vi "Print XML Recursive Priv.vi"(0 "Tree Dictionary In":variant, 1 "Recursion Level":i32, 2 "Data Types Dict":variant, 7 "Child IDs":string[](array[string]), 11 "error in":errorcluster, 12 "Include Type Attribute":bool=TRUE) -> (4 "Tree Dictionary Out":variant, 8 "XML String":string, 15 "error out":errorcluster)   [LabVIEW 2020, in "NI_VIAnCFGDataStructure.lvlib" / "Tree.lvclass"]
uses:
  <vilib>/addons/analyzer/VIAnCFGDataStructure/Tree Manager/Tree.lvclass
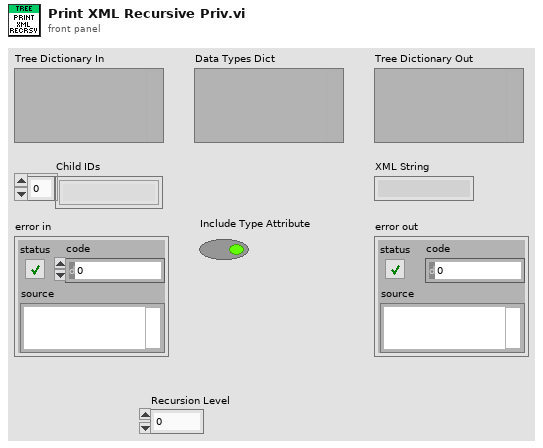
[diagram p1: front panel]
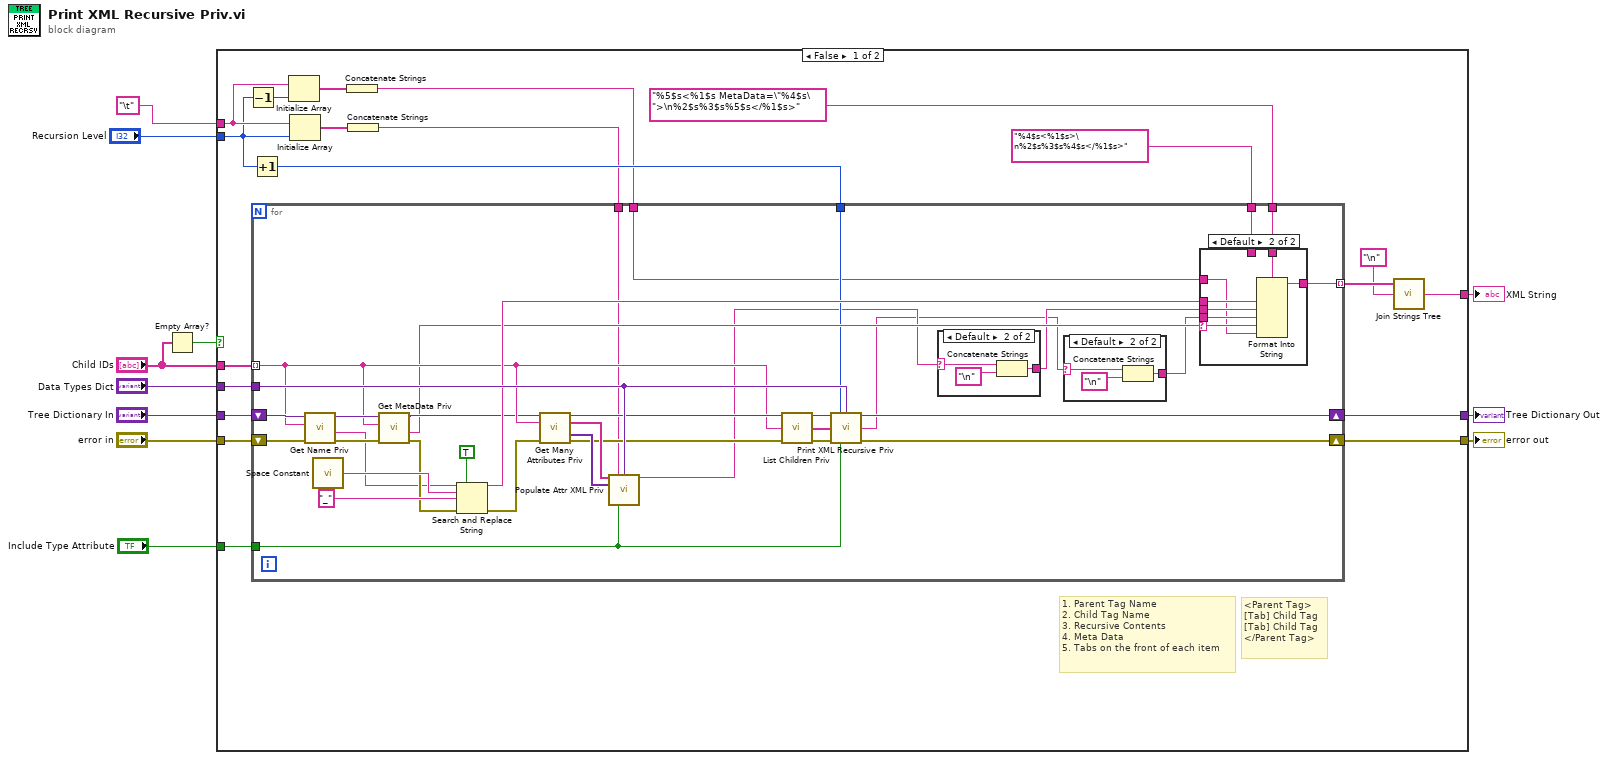
[diagram p0: block diagram]
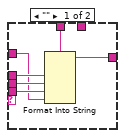
[diagram p4: hidden frame]
diagram:
  n1 = Empty Array?(array="Child IDs") -> (empty?=w1:bool)
  n2 = case shown="False" w1 {
    tunnel: [w31 w88] -> w11
    tunnel: "error in" -> [w30 w88]
    tunnel: "Tree Dictionary In" -> [w29 w89]
    tunnel: [w28 w89] -> w8
    tunnel: "Data Types Dict" -> [w27 _]
    tunnel: "Include Type Attribute" -> [w23 _]
    tunnel: "\t" -> [w15 _]
    tunnel: "Recursion Level" -> [w13 _]
    tunnel: [w19 _] -> w3
    tunnel: "Child IDs" -> [w17 _]
    frame False {
      # "<Parent Tag>\n[Tab] Child Tag\n[Tab] Child Tag\n</Parent Tag>"
      # "1. Parent Tag Name\n2. Child Tag Name\n3. Recursive Contents\n4. Meta Data\n5. Tabs on the front of each item"
      n3 = Decrement(x=w13) -> (x-1=w14:i32)
      n4 = Increment(x=w13) -> (x+1=w21:i32)
      n5 = Initialize Array(w15, w14) -> (w16:string[])
      n6 = Initialize Array(w15, w13) -> (w22:string[])
      n7 = Concatenate Strings(w16) -> (w12:string)
      n8 = Concatenate Strings(w22) -> (w20:string)
      n9 = for {
        tunnel: w17 -> [w47] mode=indexing
        shift-right: [w63] -> w28
        shift-left: w29 -> [w66]
        shift-right: [w53] -> w31
        shift-left: w30 -> [w65]
        tunnel: w27 -> [w61]
        tunnel: [w40] -> w26 mode=indexing
        tunnel: "%5$s<%1$s MetaData=\"%4$s\">\n%2$s%3$s%5$s</%1$s>" ("format string") -> [w43]
        tunnel: "%4$s<%1$s>\n%2$s%3$s%4$s</%1$s>" ("format string") -> [w42]
        tunnel: w23 -> [w41]
        tunnel: w21 -> [w39]
        tunnel: w20 -> [w32]
        tunnel: w12 -> [w33]
        n10 = call <vilib>:"Get Name Priv.vi"("error in"=w65, "Unique ID"=w47, "Tree Dictionary"=w66) -> ("error out"=w48:errorcluster, "Name"=w37:string, "Tree Dictionary Out"=w49:variant)  [unwired: 6 in]
        n11 = call <vilib>:"Space Constant.vi"() -> ("String"=w58:string)
        n12 = call <vilib>:"Get MetaData Priv.vi"("error in"=w48, "Unique ID"=w47, "Tree Dictionary"=w49) -> ("error out"=w45:errorcluster, "MetaData"=w44:string, "Tree Dictionary Out"=w46:variant)  [unwired: 6 in]
        n13 = Search and Replace String(replace all?=TRUE ("replace all? (F)"), input string=w37, search string=w58, replace string="_", error in=w45) -> (result string=w55:string, error out=w54:errorcluster)  [unwired: 3 in, 2 out]
        n14 = call <vilib>:"Get Many Attributes Priv.vi"("Tree Dictionary In"=w46, "Unique ID"=w47, "error in"=w54) -> ("Tree Dictionary Out"=w59:variant, "Attribute Names"=w52:string[], "Attribute Values"=w51:variant[], "error out"=w50:errorcluster)  [unwired: 8 in, 1 out]
        n15 = call <vilib>:"Populate Attr XML Priv.vi"("Attribute Names"=w52, "Tab String"=w32, "Data Types Dict"=w61, "Attribute Values"=w51, "Include Type Attribute"=w41) -> ("Attr XML String"=w38:string)  [unwired: 10 in]
        n16 = call <vilib>:"List Children Priv.vi"("Tree Dictionary"=w59, "Parent ID"=w47, "Error In"=w50) -> ("Tree Dictionary Out"=w64:variant, "Child IDs"=w62:string[], "Error Out"=w60:errorcluster)  [unwired: 10 in]
        n17 = call <vilib>:"Print XML Recursive Priv.vi"("Tree Dictionary In"=w64, "Recursion Level"=w39, "Data Types Dict"=w61, "Child IDs"=w62, "error in"=w60, "Include Type Attribute"=w41) -> ("Tree Dictionary Out"=w63:variant, "XML String"=w35:string, "error out"=w53:errorcluster)  [unwired: 7 in]
        n18 = case shown="Default" w38 {
          selector: w38 -> [w71 w74]
          tunnel: [w71 w73] -> w36
          frame "" {
          }
          frame Default {
            n19 = Concatenate Strings(w74, "\n") -> (w73:string)
          }
        }
        n20 = case shown="Default" w35 {
          selector: w35 -> [w67 w70]
          tunnel: [w67 w69] -> w34
          frame "" {
          }
          frame Default {
            n21 = Concatenate Strings(w70, "\n") -> (w69:string)
          }
        }
        n22 = case shown="Default" w44 {
          selector: w44 -> [_ w83]
          tunnel: [w76 w87] -> w40
          tunnel: w34 -> [w78 w86]
          tunnel: w36 -> [w79 w85]
          tunnel: w55 -> [w80 w84]
          tunnel: w43 -> [_ w82]
          tunnel: w42 -> [w77 _]
          tunnel: w33 -> [w75 w81]
          frame "" {
            n23 = Format Into String(format string=w77, w80, w79, w78, w75) -> (resulting string=w76:string)  [unwired: 2 in, 1 out]
          }
          frame Default {
            n24 = Format Into String(format string=w82, w84, w85, w86, w83, w81) -> (resulting string=w87:string)  [unwired: 2 in, 1 out]
          }
        }
      }
      n25 = call <vilib>:"Join Strings Tree.vi"("Separator (,)"="\n", "Strings In"=w26) -> ("String"=w19:string)  [unwired: 1 in]
    }
    frame True {
    }
  }
  "error out" <- w11
  "Tree Dictionary Out" <- w8
  "XML String" <- w3
